vi "Main.vi"(11 "Module Admin":refnum<class "Delacor_lib_QMH_Module Admin.lvclass">) -> ()   [LabVIEW 2024, in "Sing.lvlib"]
doc: "This template is based off of the Queued Message Handler design pattern and the Queued Message Handler project template that ships with LabVIEW.\n\nThe main difference is that the queue is private to this module and communication between modules is performed via Broadcast and Request events.\n\nRequest events are wrapped in public API methods and are handled in the Event Handling Loop (EHL) of this VI. Any module can register for Broadcast events sent by this module. The EHL generates messages based on user interface actions.\n\nThe Message Handling Loop (MHL) processes messages generated by the EHL, or by other messages. The messages are string values, so new messages can be added easily to the Message Cases case structure in the MHL. Each message cluster can also provide an optional value for Message Data, which is a variant that can be converted to whatever message-specific data is required.\n_____\nBased on DQMH Dev Tools: Project Template 7.1.0.1503."
uses:
  Sing.lvlib
  <vilib>/Delacor/Delacor QMH/Libraries/Module Admin_class/Delacor_lib_QMH_Module Admin.lvclass
  Module Data--cluster.ctl
  Do Something Argument--cluster.ctl
  <vilib>/Delacor/Delacor QMH/Libraries/Message Queue_class/Delacor_lib_QMH_Message Queue.lvclass/Delacor_lib_QMH_Message Queue.ctl
  Do Something Else Argument--cluster.ctl
  Do Something Else and Wait for Reply Argument--cluster.ctl
  Do Something Else and Wait (Reply Payload)--cluster.ctl
  Stop Argument--cluster.ctl
  <vilib>/Delacor/Delacor QMH/Libraries/Module Admin_class/Delacor_lib_QMH_Module Admin.lvclass/Delacor_lib_QMH_Module Admin.ctl
  Change FP Color Argument--cluster.ctl
  <vilib>/Delacor/Delacor QMH/Libraries/Message Queue_class/Delacor_lib_QMH_Enqueue Message (Single).vi
  <vilib>/Delacor/Delacor QMH/Libraries/Module Admin_class/Delacor_lib_QMH_Get External Launch.vi
  <vilib>/Delacor/Delacor QMH/Libraries/Message Queue_class/Delacor_lib_QMH_Message Queue.lvclass
  Cambia de colores los paneles Argument--cluster.ctl
panel:
  out "X":dbl
  in  "Do Something Else <Replace Me>":bool
  in  "Do Something <Replace Me>":bool
  out "error out":errorcluster
  out "Status":string
  in  "Simulate MHL Error":bool
  in  "Simulate EHL Error":bool
  # "These controls have associated \"Value Changed\" events configured in the Event Structure on the diagram.\n\nReplace them (and reconfigure the Event Structure) with the controls you need for your application. \n\nOther processes communicate with this Module via its Public API (wrappers for its Request Events).\n\nThis Module communicates with other processes via its Broadcast Events.\nAny process that wants to receive these messages can register for this module's Broadcast events."
  # "This template is for the DQMH framework. See the block diagram for more information on how to use this template."
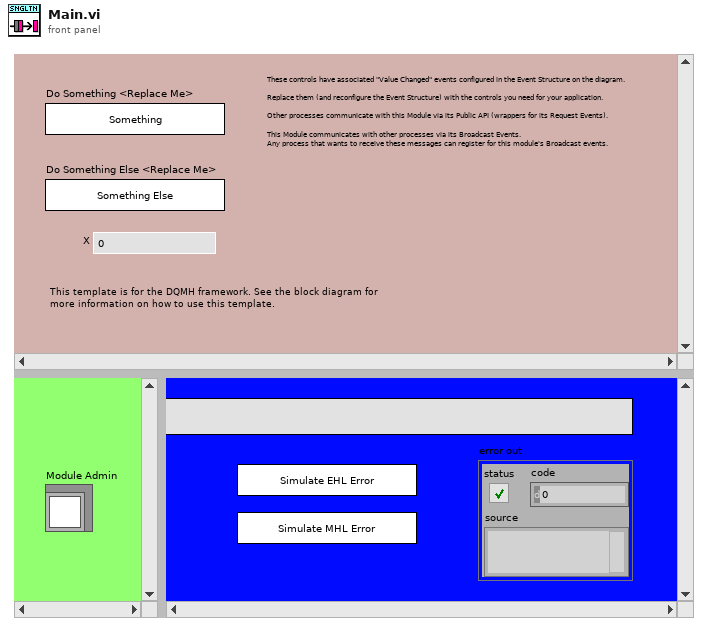
[diagram p1: front panel]
types:
  T1 = typedef "Sing.lvlib/Request Events--cluster.ctl" = cluster{"Stop Module":refnum<user-event>, "Do Something":refnum<user-event>, "Do Something Else":refnum<user-event>, "Do Something Else and Wait for Reply":refnum<user-event>, "Show Panel":refnum<user-event>, "Hide Panel":refnum<user-event>, "Get Module Execution Status":refnum<user-event>, "Show Diagram":refnum<user-event>, "Change FP Color":refnum<user-event>, "Cambia de colores los paneles":refnum<user-event>}
  T2 = typedef "Sing.lvlib/Module Data--cluster.ctl" = cluster{"Status":string}
  T3 = typedef "Sing.lvlib/Do Something Argument--cluster.ctl" = cluster{"Do Something Msg":string}
  T4 = typedef "Sing.lvlib/Do Something Else Argument--cluster.ctl" = cluster{"Do Something Else Msg":string, "X":dbl}
  T5 = typedef "Sing.lvlib/Do Something Else and Wait for Reply Argument--cluster.ctl" = cluster{"Do Something Else Msg":string, "X":dbl, "Wait Notifier":refnum<notifier>, "wait for reply":bool}
  T6 = enum32{"invalid lock state", "Not Locked", "Locked (No Password)", "Password-protected"}
  T7 = typedef "Sing.lvlib/Stop Argument--cluster.ctl" = cluster{"Origin":string, "Exit via Stop Module Req?":bool, "Wait for Module to stop?":bool}
  T8 = typedef "Sing.lvlib/Change FP Color Argument--cluster.ctl" = cluster{"FP Color":u32[]}
  T9 = typedef "Sing.lvlib/Cambia de colores los paneles Argument--cluster.ctl" = cluster{"Colores":u32[]}
  T10 = enum32{"Invalid", "Standard", "Closed", "Hidden", "Minimized", "Maximized"}
  T11 = typedef "Sing.lvlib/Do Something Else and Wait (Reply Payload)--cluster.ctl" = cluster{"Value":dbl, "error":errorcluster}
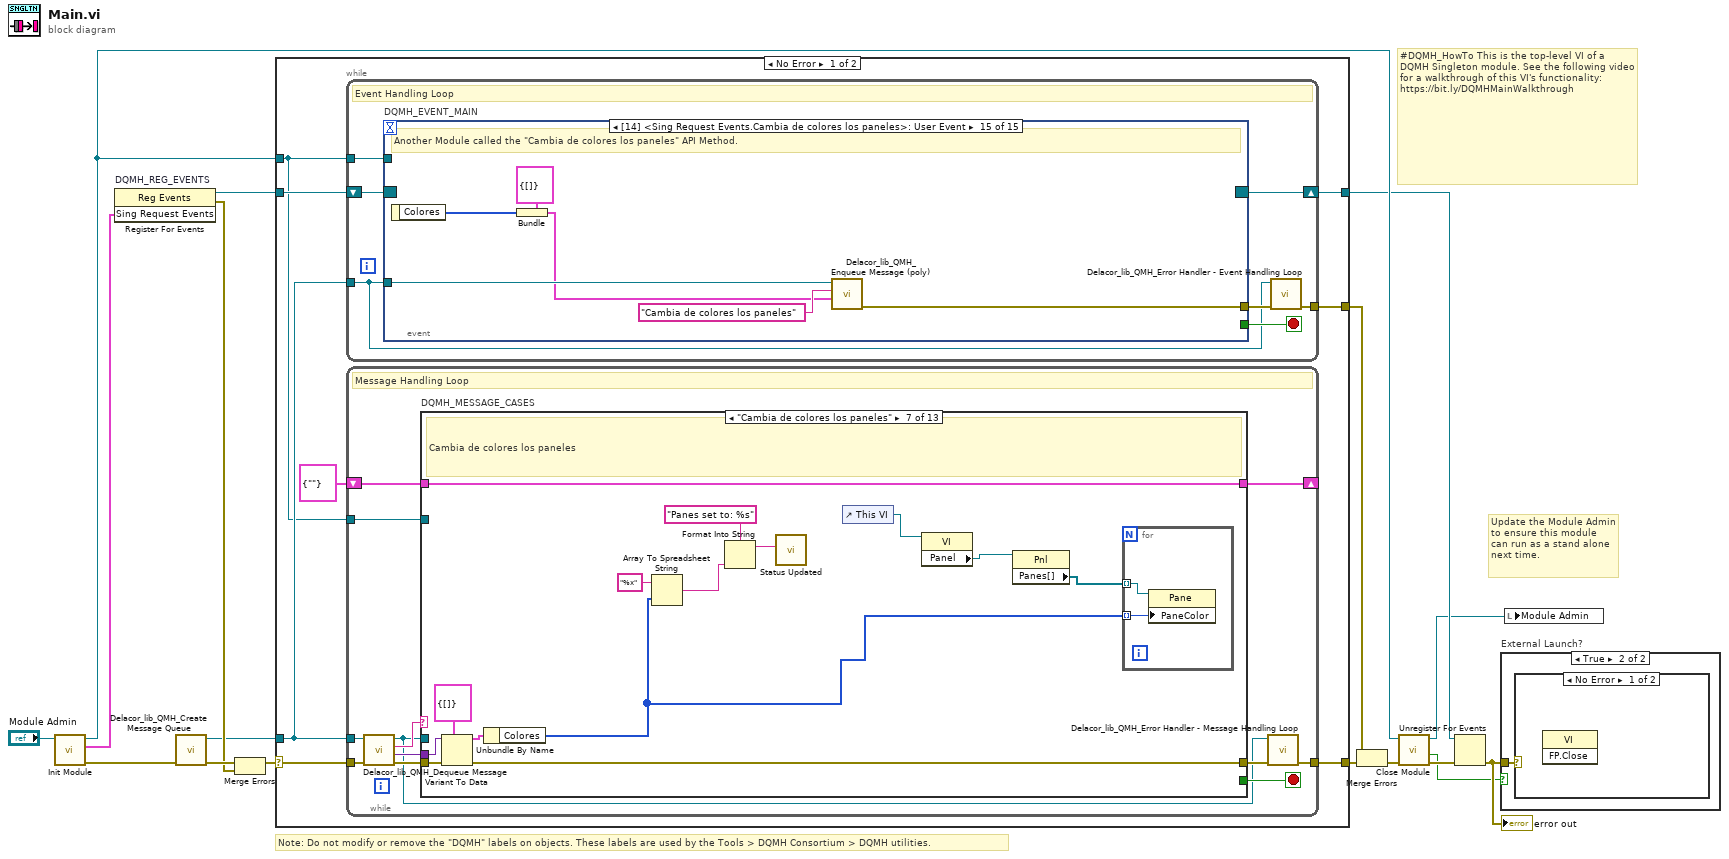
[diagram p0: block diagram]
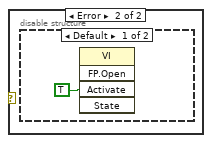
[diagram p3: hidden frame]
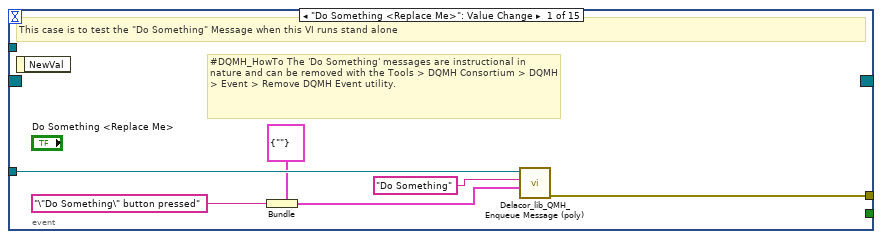
[diagram p5: hidden frame]
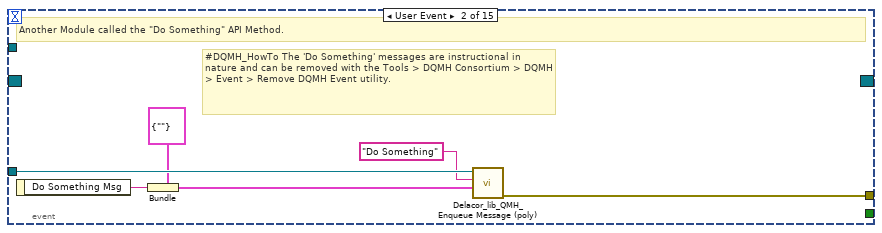
[diagram p6: hidden frame]
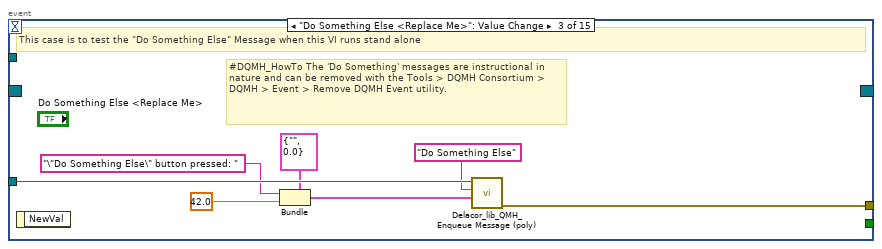
[diagram p7: hidden frame]
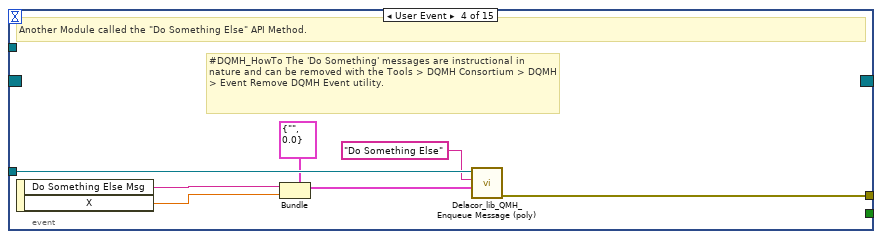
[diagram p8: hidden frame]
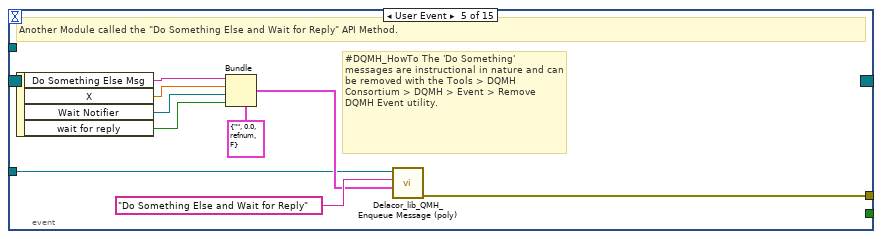
[diagram p9: hidden frame]
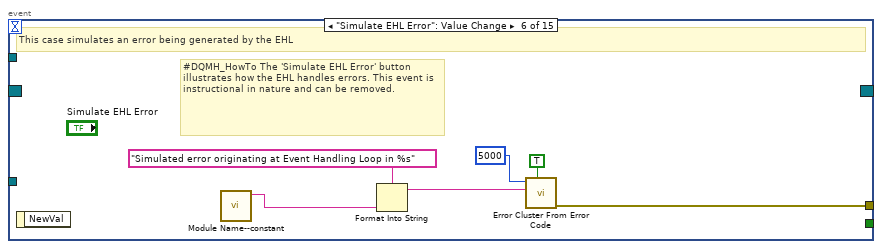
[diagram p10: hidden frame]
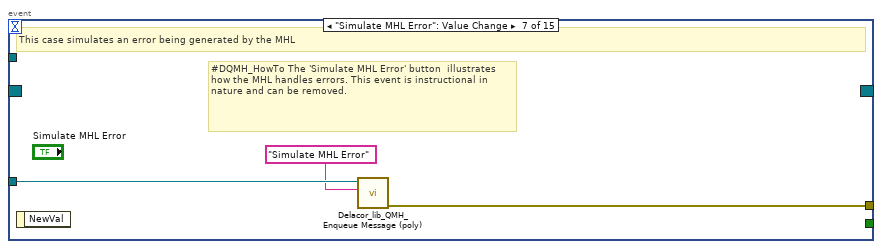
[diagram p11: hidden frame]
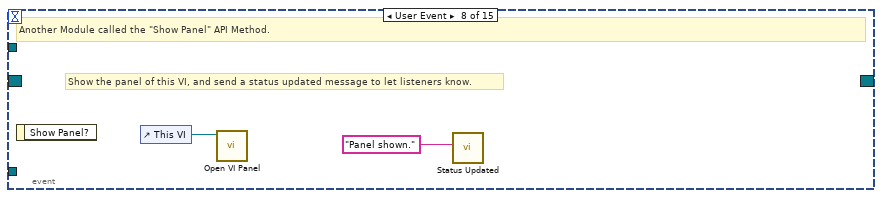
[diagram p12: hidden frame]
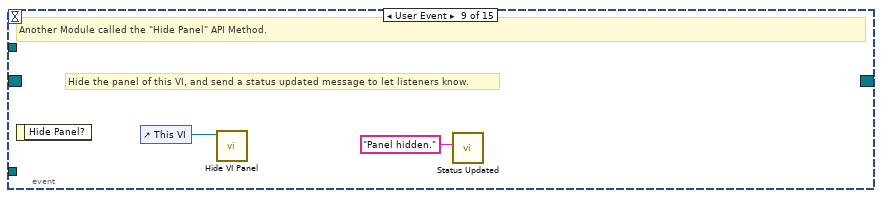
[diagram p13: hidden frame]
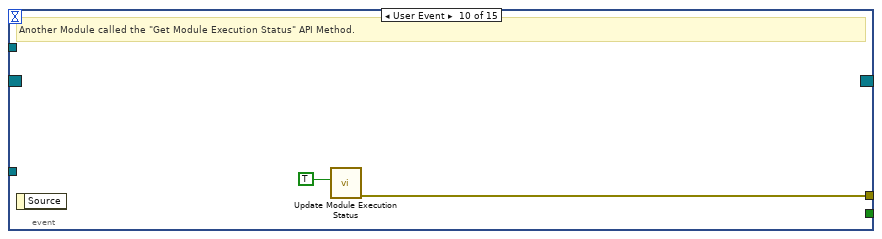
[diagram p14: hidden frame]
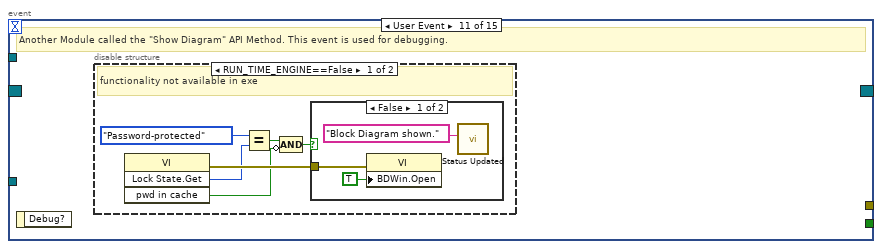
[diagram p15: hidden frame]
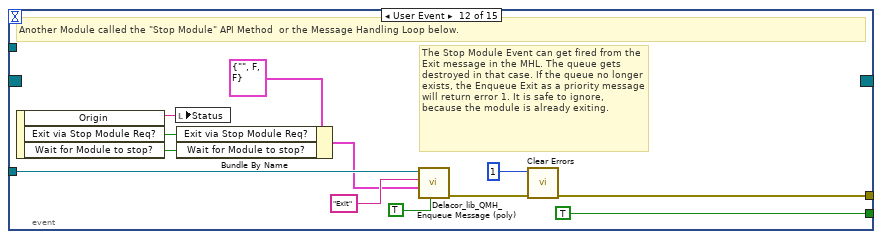
[diagram p18: hidden frame]
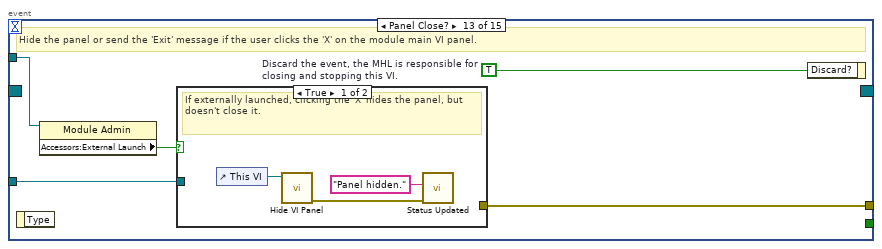
[diagram p19: hidden frame]
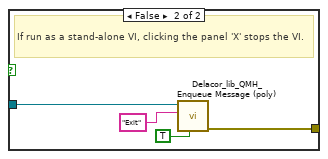
[diagram p20: hidden frame]
diagram:
  # "#DQMH_HowTo This is the top-level VI of a DQMH Singleton module. See the following video for a walkthrough of this VI's functionality: https://bit.ly/DQMHMainWalkthrough"
  # "Note: Do not modify or remove the \"DQMH\" labels on objects. These labels are used by the Tools > DQMH Consortium > DQMH utilities."
  # "Update the Module Admin to ensure this module can run as a stand alone next time."
  n1 = call "Init Module.vi"("Singleton Module Admin in"="Module Admin") -> ("error out"=w16:errorcluster, "Sing Request Events"=w5:T1, "Singleton Module Admin out"=w8:refnum<class "Delacor_lib_QMH_Module Admin.lvclass">)  [unwired: 8 in]
  n2 = register-events "DQMH_REG_EVENTS"(w5) -> (reference out=w6:refnum<event-registration>, error out=w9:errorcluster)  [unwired: 2 in]
  n3 = call <vilib>:"Delacor_lib_QMH_Create Message Queue.vi"("error in"=w16) -> ("error out"=w11:errorcluster, "Message Queue"=w4:refnum<class "Delacor_lib_QMH_Message Queue.lvclass">)  [unwired: 9 in]
  n4 = Merge Errors(w11, w9) -> (w10:errorcluster)
  n5 = case shown="No Error" w10 {
    selector: w10 -> [w23 w302]
    tunnel: [w25 w301] -> w17
    tunnel: [w22 w300] -> w7
    tunnel: w6 -> [w20 w300]
    tunnel: w4 -> [w19 w295]
    tunnel: [w24 _] -> w14
    tunnel: w8 -> [w18 w296]
    frame No Error {
      n6 = while {
        tunnel: w19 -> [w26]
        shift-right: [w29] -> w22
        shift-left: w20 -> [w30]
        tunnel: [w31] -> w24
        tunnel: w18 -> [w27]
        stop <- w28 stop-if-true
        # "Event Handling Loop"
        n7 = event "DQMH_EVENT_MAIN" shown="[14] <Sing Request Events.Cambia de colores los paneles>: User Event" {
          selector: w30 -> [_ _ _ _ _ _ _ _ _ _ _ _ _ _ _]
          dyn-events: [_ _ _ _ _ _ _ _ _ _ _ _ _ _ _] -> w29
          timeout: _ -> [_ _ _ _ _ _ _ _ _ _ _ _ _ _ _]
          tunnel: [_ _ _ _ _ _ _ _ _ _ _ TRUE ("Discard?") _ _ _] -> w28
          tunnel: w26 -> [w37 w43 w50 w57 w60 _ w75 _ _ _ _ w99 w106 w121 w127]
          tunnel: [w38 w44 w51 w58 w67 w73 w76 _ _ w82 _ w102 w108 w116 w122] -> w32
          tunnel: w27 -> [_ _ _ _ _ _ _ _ _ _ _ _ w105 _ _]
          event "Do Something <Replace Me>": Value Change {
            # "#DQMH_HowTo The 'Do Something' messages are instructional in nature and can be removed with the Tools > DQMH Consortium > DQMH > Event > Remove DQMH Event utility."
            # "This case is to test the \"Do Something\" Message when this VI runs stand alone"
            n8 = event-data() -> ()  [unwired: 1 in, 1 out]
            n9 = Bundle(cluster=T3 {"Do Something Msg"=""} ("Do Something Argument"), "Do Something Msg"="\"Do Something\" button pressed" ("\"Do Something\" button pressed")) -> (w33:T3)
            n10 = call-poly <vilib>:"Delacor_lib_QMH_Enqueue Message (poly).vi"("Message Data"=w33, "Message"="Do Something", "Message Queue in"=w37) -> ("error out"=w38:errorcluster)  [unwired: 7 in, 1 out]
          }
          event User Event {
            # "#DQMH_HowTo The 'Do Something' messages are instructional in nature and can be removed with the Tools > DQMH Consortium > DQMH > Event > Remove DQMH Event utility."
            # "Another Module called the \"Do Something\" API Method."
            n11 = event-data() -> ("Do Something Msg"=w40:string)  [unwired: 1 in]
            n12 = Bundle(cluster=T3 {"Do Something Msg"=""} ("Do Something Argument"), "Do Something Msg"=w40) -> (w39:T3)
            n13 = call-poly <vilib>:"Delacor_lib_QMH_Enqueue Message (poly).vi"("Message Data"=w39, "Message"="Do Something", "Message Queue in"=w43) -> ("error out"=w44:errorcluster)  [unwired: 7 in, 1 out]
          }
          event "Do Something Else <Replace Me>": Value Change {
            # "#DQMH_HowTo The 'Do Something' messages are instructional in nature and can be removed with the Tools > DQMH Consortium > DQMH > Event > Remove DQMH Event utility."
            # "This case is to test the \"Do Something Else\" Message when this VI runs stand alone"
            n14 = event-data() -> ()  [unwired: 1 in, 1 out]
            n15 = Bundle(cluster=T4 {"Do Something Else Msg"="", "X"=0.0} ("Do Something Else Argument"), "Do Something Else Msg"="\"Do Something Else\" button pressed: " ("\"Do Something Else\" button pressed"), "X"=42.0) -> (w47:T4)
            n16 = call-poly <vilib>:"Delacor_lib_QMH_Enqueue Message (poly).vi"("Message Data"=w47, "Message"="Do Something Else", "Message Queue in"=w50) -> ("error out"=w51:errorcluster)  [unwired: 7 in, 1 out]
          }
          event User Event {
            # "#DQMH_HowTo The 'Do Something' messages are instructional in nature and can be removed with the Tools > DQMH Consortium > DQMH > Event Remove DQMH Event utility."
            # "Another Module called the \"Do Something Else\" API Method."
            n17 = event-data() -> ("Do Something Else Msg"=w53:string, "X"=w52:dbl)  [unwired: 1 in]
            n18 = Bundle(cluster=T4 {"Do Something Else Msg"="", "X"=0.0} ("Do Something Else Argument"), "Do Something Else Msg"=w53, "X"=w52) -> (w54:T4)
            n19 = call-poly <vilib>:"Delacor_lib_QMH_Enqueue Message (poly).vi"("Message Data"=w54, "Message"="Do Something Else", "Message Queue in"=w57) -> ("error out"=w58:errorcluster)  [unwired: 7 in, 1 out]
          }
          event User Event {
            # "#DQMH_HowTo The 'Do Something' messages are instructional in nature and can be removed with the Tools > DQMH Consortium > DQMH > Event > Remove DQMH Event utility."
            # "Another Module called the \"Do Something Else and Wait for Reply\" API Method."
            n20 = event-data() -> ("Do Something Else Msg"=w63:string, "X"=w62:dbl, "Wait Notifier"=w61:refnum<notifier>, "wait for reply"=w59:bool)  [unwired: 1 in]
            n21 = Bundle(cluster=T5 {"Do Something Else Msg"="", "X"=0.0, "Wait Notifier"=refnum, "wait for reply"=FALSE} ("Do Something Else and Wait for Reply Argument"), "Do Something Else Msg"=w63, "X"=w62, "Wait Notifier"=w61, "wait for reply"=w59) -> (w64:T5)
            n22 = call-poly <vilib>:"Delacor_lib_QMH_Enqueue Message (poly).vi"("Message Data"=w64, "Message"="Do Something Else and Wait for Reply", "Message Queue in"=w60) -> ("error out"=w67:errorcluster)  [unwired: 7 in, 1 out]
          }
          event "Simulate EHL Error": Value Change {
            # "#DQMH_HowTo The 'Simulate EHL Error' button  illustrates how the EHL handles errors. This event is instructional in nature and can be removed."
            # "This case simulates an error being generated by the EHL"
            n23 = event-data() -> ()  [unwired: 1 in, 1 out]
            n24 = call "Module Name--constant.vi"() -> ("Module Name"=w70:string)  [unwired: 11 in]
            n25 = Format Into String(format string="Simulated error originating at Event Handling Loop in %s", w70) -> (resulting string=w71:string)  [unwired: 2 in, 1 out]
            n26 = call <vilib>:"Error Cluster From Error Code.vi"("show call chain? (False)"=TRUE, "error message (\"\")"=w71, "error code (0)"=5000) -> ("error out"=w73:errorcluster)  [unwired: 6 in]
          }
          event "Simulate MHL Error": Value Change {
            # "#DQMH_HowTo The 'Simulate MHL Error' button  illustrates how the MHL handles errors. This event is instructional in nature and can be removed."
            # "This case simulates an error being generated by the MHL"
            n27 = event-data() -> ()  [unwired: 1 in, 1 out]
            n28 = call-poly <vilib>:"Delacor_lib_QMH_Enqueue Message (poly).vi"("Message"="Simulate MHL Error", "Message Queue in"=w75) -> ("error out"=w76:errorcluster)  [unwired: 8 in, 1 out]
          }
          event User Event {
            # "Show the panel of this VI, and send a status updated message to let listeners know."
            # "Another Module called the \"Show Panel\" API Method."
            n29 = event-data() -> ()  [unwired: 1 in, 1 out]
            n30 = control-ref of="This VI"() -> (w78:refnum<vi>)
            n31 = call "Open VI Panel.vi"("VI"=w78) -> ()  [unwired: 10 in, 1 out]
            n32 = call "Status Updated.vi"("Status"="Panel shown." ("format string")) -> ()  [unwired: 10 in, 1 out]
          }
          event User Event {
            # "Hide the panel of this VI, and send a status updated message to let listeners know."
            # "Another Module called the \"Hide Panel\" API Method."
            n33 = event-data() -> ()  [unwired: 1 in, 1 out]
            n34 = control-ref of="This VI"() -> (w80:refnum<vi>)
            n35 = call "Hide VI Panel.vi"("VI"=w80) -> ()  [unwired: 10 in, 1 out]
            n36 = call "Status Updated.vi"("Status"="Panel hidden." ("format string")) -> ()  [unwired: 10 in, 1 out]
          }
          event User Event {
            # "Another Module called the \"Get Module Execution Status\" API Method."
            n37 = event-data() -> ()  [unwired: 1 in, 1 out]
            n38 = call "Update Module Execution Status.vi"("Running?"=TRUE) -> ("error out"=w82:errorcluster)  [unwired: 10 in]
          }
          event User Event {
            # "Another Module called the \"Show Diagram\" API Method. This event is used for debugging."
            n39 = event-data() -> ()  [unwired: 1 in, 1 out]
            n40 = disable-structure shown="RUN_TIME_ENGINE==False" {
              frame condition #0 (active) {
                # "functionality not available in exe"
                n41 = invoke on="Invoke Node" class="VI" method="Lock State.Get"() -> (error out=w88:errorcluster, "Get Lock State"=w87:T6, "pwd in cache"=w84:bool)  [unwired: 4 in, 1 out]
                n42 = Equal?(x=T6."Password-protected", y=w87) -> (x = y?=w85:bool)
                n43 = Compound Arithmetic op=AND(w85, invert w84) -> (w83:bool)
                n44 = case shown="False" w83 {
                  tunnel: w88 -> [w91 _]
                  frame False {
                    n45 = property on="Property Node" class="VI"(error in=w91, "BDWin.Open"=TRUE ("Block Diagram Window:Open")) -> ()  [unwired: 1 in, 2 out]
                    n46 = call "Status Updated.vi"("Status"="Block Diagram shown." ("format string")) -> ()  [unwired: 10 in, 1 out]
                  }
                  frame True {
                    # "Password-protected VI, and the password is not in the cache. Do not show the diagram."
                  }
                }
              }
              frame condition #1 {
              }
            }
          }
          event User Event {
            # "The Stop Module Event can get fired from the Exit message in the MHL. The queue gets destroyed in that case. If the queue no longer exists, the Enqueue Exit as a priority message will return error 1. It is safe to ignore, because the module is already exiting."
            # "Another Module called the \"Stop Module\" API Method  or the Message Handling Loop below."
            n47 = event-data() -> ("Origin"=w98:string, "Exit via Stop Module Req?"=w94:bool, "Wait for Module to stop?"=w93:bool)  [unwired: 1 in]
            n48 = local write "Status"(w98) -> ()
            n49 = Bundle By Name(cluster=T7 {"Origin"="", "Exit via Stop Module Req?"=FALSE, "Wait for Module to stop?"=FALSE} ("Stop Argument"), "Exit via Stop Module Req?"=w94, "Wait for Module to stop?"=w93) -> (w92:T7)
            n50 = call-poly <vilib>:"Delacor_lib_QMH_Enqueue Message (poly).vi"("Priority Message? (F)"=TRUE, "Message Data"=w92, "Message"="Exit", "Message Queue in"=w99) -> ("error out"=w103:errorcluster)  [unwired: 6 in, 1 out]
            n51 = call <vilib>:"Clear Errors.vi"("error in (no error)"=w103, "specific error code to clear (0: all)"=1) -> ("error out"=w102:errorcluster)  [unwired: 4 in, 1 out]
          }
          event Panel Close? {
            w107 = TRUE  # Discard the event, the MHL is responsible for closing and stopping this VI.
            # "Hide the panel or send the 'Exit' message if the user clicks the 'X' on the module main VI panel."
            n52 = event-data() -> ()  [unwired: 1 in, 1 out]
            n53 = property on="Property Node" class="Module Admin"(reference=w105) -> ("Accessors:External Launch"=w104:bool)  [unwired: 1 in, 2 out]
            n54 = case shown="True" w104 {
              tunnel: w106 -> [_ w114]
              tunnel: [_ w115] -> w108
              frame True {
                # "If externally launched, clicking the 'X' hides the panel, but doesn't close it."
                n55 = control-ref of="This VI"() -> (w111:refnum<vi>)
                n56 = call "Hide VI Panel.vi"("VI"=w111) -> ("error out"=w109:errorcluster)  [unwired: 10 in]
                n57 = call "Status Updated.vi"("error in"=w109, "Status"="Panel hidden." ("format string")) -> ()  [unwired: 9 in, 1 out]
              }
              frame False {
                # "If run as a stand-alone VI, clicking the panel 'X' stops the VI."
                n58 = call-poly <vilib>:"Delacor_lib_QMH_Enqueue Message (poly).vi"("Priority Message? (F)"=TRUE, "Message"="Exit", "Message Queue in"=w114) -> ("error out"=w115:errorcluster)  [unwired: 7 in, 1 out]
              }
            }
            n59 = event-data ("Event Filter Node")("Discard?"=w107) -> ()  [unwired: 1 in, 1 out]
          }
          event User Event {
            # "Another Module called the \"Change FP Color\" API Method."
            n60 = event-data() -> ("FP Color"=w117:u32[])  [unwired: 1 in]
            n61 = Bundle(cluster=T8 {"FP Color"=[]} ("Change FP Color Argument"), "FP Color"=w117) -> (w118:T8)
            n62 = call-poly <vilib>:"Delacor_lib_QMH_Enqueue Message (poly).vi"("Message Data"=w118, "Message"="Change FP Color", "Message Queue in"=w121) -> ("error out"=w116:errorcluster)  [unwired: 7 in, 1 out]
          }
          event User Event {
            # "Another Module called the \"Cambia de colores los paneles\" API Method."
            n63 = event-data() -> ("Colores"=w123:u32[])  [unwired: 1 in]
            n64 = Bundle(cluster=T9 {"Colores"=[]} ("Cambia de colores los paneles Argument"), "Colores"=w123) -> (w124:T9)
            n65 = call-poly <vilib>:"Delacor_lib_QMH_Enqueue Message (poly).vi"("Message Data"=w124, "Message"="Cambia de colores los paneles", "Message Queue in"=w127) -> ("error out"=w122:errorcluster)  [unwired: 7 in, 1 out]
          }
        }
        n66 = call-dynamic "Delacor_lib_QMH_Error Handler - Event Handling Loop.vi"("error in"=w32, "Message Queue in"=w26) -> ("dup error in"=w31:errorcluster)  [unwired: 8 in, 1 out]
      }
      n67 = while {
        tunnel: w19 -> [w128]
        shift-right: [w136] -> _
        shift-left: T2 {"Status"=""} ("Data Cluster") -> [w137]
        tunnel: w23 -> [w139]
        tunnel: [w131] -> w25
        tunnel: w18 -> [w132]
        stop <- w135 stop-if-true
        # "Message Handling Loop"
        n68 = call-dynamic "Delacor_lib_QMH_Dequeue Message.vi"("error in"=w139, "Message Queue in"=w128) -> ("error out"=w138:errorcluster, "Message Data"=w133:variant, "Message"=w134:string, "Message Queue out"=w129:refnum<class "Delacor_lib_QMH_Message Queue.lvclass">)  [unwired: 6 in]
        n69 = case "DQMH_MESSAGE_CASES" shown="\"Cambia de colores los paneles\"" w134 {
          selector: w134 -> [_ _ _ _ _ _ _ _ _ _ _ _ w290]
          tunnel: w129 -> [_ _ _ _ _ _ _ _ _ _ w256 w278 _]
          tunnel: w138 -> [w156 w160 w168 w177 w196 w220 w236 w241 w243 w252 w263 w284 w293]
          tunnel: [w154 w160 w166 w176 w195 w218 w234 w240 w243 w251 w259 w279 w294] -> w130
          tunnel: w137 -> [w145 w159 w165 w175 w192 w219 w235 w239 w242 w249 w258 w277 w291]
          tunnel: [w144 w159 w165 w175 w192 w219 w235 w239 w242 w249 w258 w277 w291] -> w136
          tunnel: [_ _ _ _ _ _ _ _ _ _ _ w276 _] -> w135
          tunnel: w133 -> [_ _ w164 w172 w189 w217 w233 _ _ _ w257 w275 _]
          tunnel: w132 -> [w146 _ _ _ _ _ _ _ _ _ w255 w270 _]
          frame "Initialize" {
            w140 = "Initial Message" ("Initial Message")
            # "#DQMH_CodeNeeded - Initialize the appearance of the front panel."
            # "#DQMH_CodeNeeded - Initialize your state data here."
            # "Initialize - Any operation that needs to be done before the module can receive messages. Synchronize Caller Events.vi will inform Start Module.vi that the module has launched and is ready to receive messages. Module Did Init.vi will broadcast that the module initialized."
            n70 = call "Synchronize Caller Events.vi"("error in"=w156, "Singleton Module Admin in"=w146) -> ("error out"=w155:errorcluster, "Singleton Module Admin out"=w141:refnum<class "Delacor_lib_QMH_Module Admin.lvclass">)  [unwired: 8 in]
            n71 = property on="Property Node" class="Module Admin"(reference=w141) -> ("Accessors:External Launch"=w150:bool)  [unwired: 1 in, 2 out]
            n72 = Select(t=T10."Hidden" ("State"), s=w150, f=T10."Standard" ("State")) -> (s? t:f=w147:T10)
            n73 = call "Module Name--constant.vi"() -> ("Module Name"=w153:string)  [unwired: 11 in]
            n74 = property on="Property Node" class="VI"("Front Panel.Title"=w153) -> (reference out=w152:refnum<vi>, error out=w158:errorcluster)  [unwired: 2 in]
            n75 = invoke on="Invoke Node" class="VI" method="FP.Open"(reference=w152, error in=w158, "State"=w147) -> (reference out=w151:refnum<vi>, error out=w157:errorcluster)  [unwired: 2 in, 3 out]
            n76 = Bundle By Name(cluster=w145, "Status"=w140) -> (w144:T2)
            n77 = invoke on="Invoke Node" class="VI" method="FP.Center"(reference=w151, error in=w157) -> ()  [unwired: 1 in, 3 out]
            n78 = call "Module Name--constant.vi"() -> ("Module Name"=w142:string)  [unwired: 11 in]
            n79 = call "Module Did Init.vi"("error in"=w155, "Initialized?"=TRUE, "Origin"=w142) -> ("error out"=w154:errorcluster)  [unwired: 8 in]
            "Status" <- w140
          }
          frame "---Module Specific---" {
            # "Separator -- The following cases handle messages specific to this Module."
          }
          frame "Do Something" {
            # "#DQMH_HowTo The 'Do Something' messages are instructional in nature and can be removed with the Tools > DQMH Consortium > DQMH > Event > Remove DQMH Event utility."
            # "Do Something - Replace this message with functionality for your own application. Note that this message also fires the \"Did Something\" broadcast event."
            n80 = Variant To Data(error in=w168, type=T3 {"Do Something Msg"=""} ("Do Something Argument"), Variant=w164) -> (data=w163:T3, error out=w167:errorcluster)
            n81 = Unbundle By Name(w163) -> ("Do Something Msg"=w161:string)
            n82 = call "Did Something.vi"("error in"=w167, "Did Something Msg"=w161) -> ("error out"=w166:errorcluster)  [unwired: 9 in]
            n83 = local write "Status"(w161) -> ()
            n84 = call "Status Updated.vi"("Status"=w161) -> ()  [unwired: 10 in, 1 out]
          }
          frame "Do Something Else" {
            # "#DQMH_HowTo The 'Do Something' messages are instructional in nature and can be removed with the Tools > DQMH Consortium > DQMH > Event > Remove DQMH Event utility."
            # "Do Something Else - Replace this message with functionality for your own application."
            n85 = Variant To Data(error in=w177, type=T4 {"Do Something Else Msg"="", "X"=0.0} ("Do Something Else Argument"), Variant=w172) -> (data=w173:T4, error out=w176:errorcluster)
            n86 = Unbundle By Name(w173) -> ("Do Something Else Msg"=w171:string, "X"=w170:dbl)
            "X" <- w170
            n87 = Format Into String(initial string=w171, w170) -> (resulting string=w169:string)  [unwired: 2 in, 1 out]
            n88 = local write "Status"(w169) -> ()
            n89 = call "Status Updated.vi"("Status"=w169) -> ()  [unwired: 10 in, 1 out]
          }
          frame "Do Something Else and Wait for Reply" {
            w184 = "X(%.2f)+Offset(%.2f)=%.2f"  # status message format string
            # "#DQMH_HowTo The 'Do Something' messages are instructional in nature and can be removed."
            # "Send back X with a random offset"
            # "Do Something Else and Wait for Reply - Replace this message with functionality for your own application. Note that this message must fire a notifier to let callers know it has finished execution, and it returns an error if the 'Value' is negative."
            n90 = Variant To Data(error in=w196, type=T5 {"Do Something Else Msg"="", "X"=0.0, "Wait Notifier"=refnum, "wait for reply"=FALSE} ("Do Something Else and Wait for Reply Argument"), Variant=w189) -> (data=w190:T5, error out=w194:errorcluster)
            n91 = Unbundle By Name(w190) -> ("Wait Notifier"=w178:refnum<notifier>, "Do Something Else Msg"=w188:string, "X"=w185:dbl, "wait for reply"=w181:bool)
            n92 = Random Number (0-1)() -> (number: 0 to 1=w186:dbl)
            n93 = Add(x=w186, y=w185) -> (x+y=w180:dbl)
            n94 = Less Than 0?(x=w180) -> (x < 0?=w183:bool)
            n95 = local write "X"(w185) -> ()
            n96 = case shown="True" w183 {
              tunnel: [_ w206] -> w193
              frame False {
              }
              frame True {
                n97 = call <vilib>:"Error Cluster From Error Code.vi"("show call chain? (False)"=TRUE, "error message (\"\")"="The 'Something Else and Wait for Reply' message generated a negative number, which is considered an error condition.", "error code (0)"=5000) -> ("error out"=w206:errorcluster)  [unwired: 6 in]
              }
            }
            n98 = Format Into String(format string=w184, initial string=w188, w185, w186, w180) -> (resulting string=w182:string)  [unwired: 1 in, 1 out]
            n99 = Bundle By Name(cluster=T11 {"Value"=0.0, "error"={"status"=FALSE, "code"=0, "source"=""}} ("notification"), "error"=w193, "Value"=w180) -> (w179:T11)
            n100 = local write "Status"(w182) -> ()
            n101 = call "Status Updated.vi"("Status"=w182) -> ()  [unwired: 10 in, 1 out]
            n102 = case shown="True" w181 {
              tunnel: w179 -> [_ w199]
              tunnel: w178 -> [_ w198]
              frame False {
              }
              frame True {
                # "Simulate an operation that requires a wait."
                n103 = flat-sequence {
                  tunnel: w199 -> [w202]
                  tunnel: w198 -> [w201]
                  tunnel: w197 -> [_]
                  frame #0 {
                    n104 = Send Notification(notification=w202, notifier=w201) -> ()  [unwired: 1 in, 2 out]
                  }
                }
                n105 = Wait (ms)(milliseconds to wait=u32 1000) -> (millisecond timer value=w197:u32)
              }
            }
            n106 = Merge Errors(w194, w193) -> (w195:errorcluster)
          }
          frame "Change FP Color" {
            n107 = Variant To Data(error in=w220, type=T8 {"FP Color"=[]} ("Change FP Color Argument"), Variant=w217) -> (data=w215:T8, error out=w218:errorcluster)
            n108 = Unbundle By Name(w215) -> ("FP Color"=w210:u32[])
            n109 = Array To Spreadsheet String(array=w210, 3:"%x" ("format string")) -> (spreadsheet string=w208:string)  [unwired: 1 in]
            n110 = Format Into String(format string="Panes set to: %s", w208) -> (resulting string=w211:string)  [unwired: 2 in, 1 out]
            n111 = call "Status Updated.vi"("Status"=w211) -> ()  [unwired: 10 in, 1 out]
            n112 = control-ref of="This VI"() -> (w214:refnum<vi>)
            n113 = property class="VI"(reference=w214) -> ("Panel"=w213:refnum<vi>)  [unwired: 1 in, 2 out]
            n114 = property class="Pnl"(reference=w213) -> ("Panes[]"=w212:refnum<vi>[])  [unwired: 1 in, 2 out]
            n115 = for {
              tunnel: w212 -> [w222] mode=indexing
              tunnel: w210 -> [w221] mode=indexing
              n116 = property class="Pane"(reference=w222, "PaneColor"=w221) -> ()  [unwired: 1 in, 2 out]
            }
          }
          frame "Cambia de colores los paneles" {
            # "Cambia de colores los paneles"
            n117 = Variant To Data(error in=w236, type=T9 {"Colores"=[]} ("Cambia de colores los paneles Argument"), Variant=w233) -> (data=w231:T9, error out=w234:errorcluster)
            n118 = Unbundle By Name(w231) -> ("Colores"=w223:u32[])
            n119 = Array To Spreadsheet String(array=w223, 3:"%x" ("format string")) -> (spreadsheet string=w225:string)  [unwired: 1 in]
            n120 = Format Into String(format string="Panes set to: %s", w225) -> (resulting string=w227:string)  [unwired: 2 in, 1 out]
            n121 = call "Status Updated.vi"("Status"=w227) -> ()  [unwired: 10 in, 1 out]
            n122 = control-ref of="This VI"() -> (w230:refnum<vi>)
            n123 = property class="VI"(reference=w230) -> ("Panel"=w229:refnum<vi>)  [unwired: 1 in, 2 out]
            n124 = property class="Pnl"(reference=w229) -> ("Panes[]"=w228:refnum<vi>[])  [unwired: 1 in, 2 out]
            n125 = for {
              tunnel: w228 -> [w238] mode=indexing
              tunnel: w223 -> [w237] mode=indexing
              n126 = property class="Pane"(reference=w238, "PaneColor"=w237) -> ()  [unwired: 1 in, 2 out]
            }
          }
          frame "---Copy This Frame---" {
            # "Duplicate this frame when creating new messages.  Change this comment in the duplicated frame to describe this message."
            n127 = Merge Errors(w241) -> (w240:errorcluster)
          }
          frame "---Exit and Error Handling---" {
            # "Separator - The following cases handle errors and exit messages."
          }
          frame "Simulate MHL Error" {
            # "#DQMH_HowTo The 'Simulate MHL Error' button  illustrates how the MHL handles errors. This event is instructional in nature and can be removed."
            # "Simulate an error occurring at the MHL"
            n128 = call "Module Name--constant.vi"() -> ("Module Name"=w245:string)  [unwired: 11 in]
            n129 = Format Into String(format string="Simulated error originating at Message Handling Loop in %s", w245) -> (resulting string=w246:string)  [unwired: 2 in, 1 out]
            n130 = call <vilib>:"Error Cluster From Error Code.vi"("show call chain? (False)"=TRUE, "error message (\"\")"=w246, "error code (0)"=5001) -> ("error out"=w250:errorcluster)  [unwired: 6 in]
            n131 = Merge Errors(w252, w250) -> (w251:errorcluster)
          }
          frame "Error" {
            # "#DQMH_CodeRecommended - If the module is running in standalone mode (External Launch = FALSE), this code will pop up an error dialog and call the 'Exit' message if an error occurs. Add more fine-grained error management here."
            # "Error - Check the error message data and respond accordingly. This message is sent by the \"Error Handler\" VIs at the end of each loop in this application."
            n132 = property on="Property Node" class="Module Admin"(reference=w255) -> ("Accessors:External Launch"=w254:bool)  [unwired: 1 in, 2 out]
            n133 = Variant To Data(error in=w263, type=errorcluster {"status"=FALSE, "code"=0, "source"=""} ("error constant"), Variant=w257) -> (data=w253:errorcluster, error out=w261:errorcluster)
            n134 = local write "error out"(w253) -> ()
            n135 = call "Error Reported.vi"("Error"=w253) -> ()  [unwired: 10 in, 1 out]
            n136 = case shown="False" w254 {
              tunnel: [w268 _] -> w260
              tunnel: w256 -> [w266 _]
              tunnel: w253 -> [w267 _]
              frame False {
                n137 = disable-structure shown="Default" {
                  disable-tunnel: w267 -> [w269 _]
                  frame condition #0 (active) {
                    # "If the module is running standalone, then pop up an error dialog and call the \"Exit\" message."
                    n138 = call <vilib>:"Simple Error Handler.vi"("error in (no error)"=w269) -> ()  [unwired: 4 in, 5 out]
                  }
                  frame condition #1 {
                    # "To prevent the Simple Error Handler VI from being loaded (e.g. when deploying to a Real-Time target), add the Conditional Disable Symbol \"DQMH_Disable_SEH\" to your project and set it to TRUE."
                  }
                }
                n139 = call-poly <vilib>:"Delacor_lib_QMH_Enqueue Message (poly).vi"("Priority Message? (F)"=TRUE, "Message"="Exit", "Message Queue in"=w266) -> ("error out"=w268:errorcluster)  [unwired: 7 in, 1 out]
              }
              frame True {
                # "If the module was launched externally, calling the Error Reported broadcast VI is the only action performed by the \"Error\" message. The module's caller can then process the error appropriately."
              }
            }
            n140 = Merge Errors(w261, w260) -> (w259:errorcluster)
          }
          frame "Exit" {
            w274 = 91  # 91: not all Exit messages will have an argument
            w276 = TRUE  # Stop the VI
            # "Release the message queue reference"
            # "#DQMH_CodeNeeded - Add any required cleanup code here."
            # "Exit - Exit the application."
            n141 = Variant To Data(error in=w284, type=T7 {"Origin"="", "Exit via Stop Module Req?"=FALSE, "Wait for Module to stop?"=FALSE} ("Stop Argument"), Variant=w275) -> (data=w272:T7, error out=w281:errorcluster)
            n142 = call <vilib>:"Clear Errors.vi"("error in (no error)"=w281, "specific error code to clear (0: all)"=w274) -> ("error out"=w283:errorcluster)  [unwired: 4 in, 1 out]
            n143 = control-ref of="This VI"() -> (w271:refnum<vi>)
            n144 = call-dynamic "Delacor_lib_QMH_Release Message Queue.vi"("error in"=w283, "Message Queue"=w278) -> ("error out"=w282:errorcluster)  [unwired: 9 in]
            n145 = call "Handle Exit.vi"("Stop Argument"=w272, "Admin in"=w270, "VI reference"=w271) -> ("error out"=w280:errorcluster)  [unwired: 7 in, 1 out]
            n146 = Merge Errors(w282, w280) -> (w279:errorcluster)
            n147 = call "Error Reported.vi"("Error"=w279) -> ()  [unwired: 10 in, 1 out]
          }
          frame Default {
            # "'Default' case only runs if there is a message that isn't defined in any of the other cases.  Output a programming error."
            n148 = call "Module Name--constant.vi"() -> ("Module Name"=w289:string)  [unwired: 11 in]
            n149 = Format Into String(format string="The invalid message string \"%s\" was received in the Message Handling Loop for module \"%s\".", w290, w289) -> (resulting string=w285:string)  [unwired: 2 in, 1 out]
            n150 = call <vilib>:"Error Cluster From Error Code.vi"("show call chain? (False)"=TRUE, "error message (\"\")"=w285, "error code (0)"=1) -> ("error out"=w292:errorcluster)  [unwired: 6 in]
            n151 = Merge Errors(w293, w292) -> (w294:errorcluster)
          }
        }
        n152 = call-dynamic "Delacor_lib_QMH_Error Handler - Message Handling Loop.vi"("error in"=w130, "Message Queue in"=w129) -> ("dup error in"=w131:errorcluster)  [unwired: 8 in, 1 out]
      }
    }
    frame Error {
      # "Synchronize Caller Events.vi will inform Start Module.vi that the module has launched and will let the code calling Start Module.vi register for broadcasts and would permit the caller receive the broadcast that an error occurred at launch time."
      n153 = call-dynamic "Delacor_lib_QMH_Release Message Queue.vi"("error in"=w302, "Message Queue"=w295) -> ("error out"=w301:errorcluster)  [unwired: 9 in]
      n154 = call "Synchronize Caller Events.vi"("Singleton Module Admin in"=w296) -> ("error out"=w303:errorcluster)  [unwired: 9 in, 1 out]
      n155 = call "Module Name--constant.vi"() -> ("Module Name"=w299:string)  [unwired: 11 in]
      n156 = Format Into String(format string="An error occurred during initialization. %s is no longer running.", w299) -> (resulting string=w297:string)  [unwired: 2 in, 1 out]
      n157 = Merge Errors(w301, w303) -> (w304:errorcluster)
      n158 = call "Error Reported.vi"("Additional Information"=w297, "Error"=w304) -> ()  [unwired: 9 in, 1 out]
    }
  }
  n159 = Merge Errors(w14, w17) -> (w13:errorcluster)
  n160 = call "Close Module.vi"("error in"=w13, "Module Admin in"=w8) -> ("error out"=w15:errorcluster, "External Launch"=w1:bool, "Module Admin out"=w2:refnum<class "Delacor_lib_QMH_Module Admin.lvclass">)  [unwired: 7 in]
  n161 = Unregister For Events(event registration refnum=w7, error in=w15) -> (error out=w12:errorcluster)
  "error out" <- w12
  n162 = case "External Launch?" shown="True" w1 {
    tunnel: w12 -> [_ w305]
    frame False {
    }
    frame True {
      n163 = case shown="No Error" w305 {
        frame No Error {
          n164 = invoke on="Invoke Node" class="VI" method="FP.Close"() -> ()  [unwired: 3 in, 3 out]
        }
        frame Error {
          n165 = disable-structure shown="Default" {
            frame condition #0 (active) {
              n166 = invoke class="VI" method="FP.Open"("Activate"=TRUE ("Activate?")) -> ()  [unwired: 4 in, 5 out]
            }
            frame condition #1 {
              # "Don't show panel on error if running inside a built EXE."
            }
          }
        }
      }
    }
  }
  n167 = local write "Module Admin"(w2) -> ()
